vi "Count delay.vi"(8 "input valid":bool=TRUE, 10 "Count to skip":u32, 11 "Reset":bool) -> (0 "output valid":bool, 2 "count done?":bool)   [LabVIEW 2013]
uses:
  Program/National Instruments/LabVIEW 2013/instr.lib/_niInstr/Basic Elements/v1/FPGA/Private/Count Down U32.vi
  Program/National Instruments/LabVIEW 2013/instr.lib/_niInstr/Basic Elements/v1/FPGA/niInstr Basic Elements v1 FPGA.lvlib
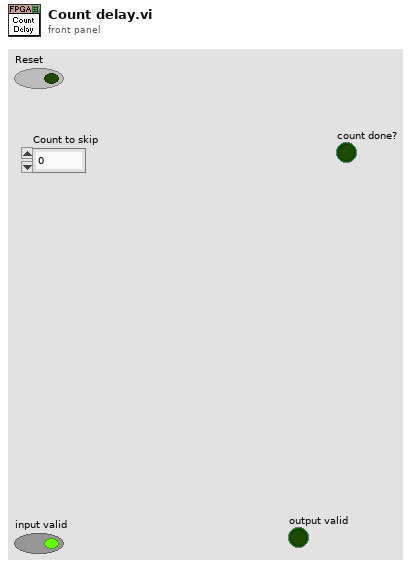
[diagram p1: front panel]
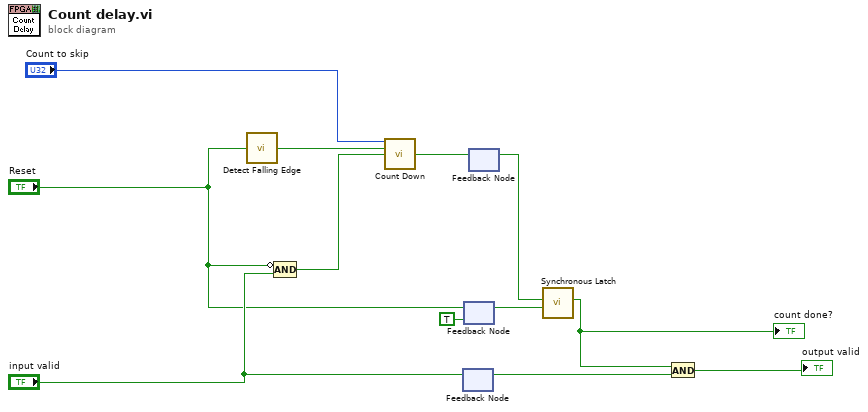
[diagram p0: block diagram]
diagram:
  n1 = call "Detect Falling Edge.vi"("signal"="Reset") -> ("edge detected"=w11:bool)  [unwired: 14 in]
  n2 = Compound Arithmetic op=AND(invert "Reset", "input valid") -> (w6:bool)
  n3 = call-poly "Count Down.vi"("count in"="Count to skip", "load"=w11, "decrement"=w6) -> ("terminal count"=w10:bool)  [unwired: 11 in, 1 out]
  n4 = feedback #1() -> (w8:bool)  [unwired: 1 in]
  n5 = feedback-in #1("input valid") -> ()
  n6 = feedback #2(TRUE) -> (w9:bool)
  n7 = feedback-in #2("Reset") -> ()
  n8 = feedback #3() -> (w5:bool)  [unwired: 1 in]
  n9 = feedback-in #3(w10) -> ()
  n10 = call "Synchronous Latch.vi"("clear"=w9, "set"=w5) -> ("out"=w4:bool)  [unwired: 9 in]
  "count done?" <- w4
  n11 = And(x=w4, y=w8) -> (x .and. y?=→"output valid":bool)
